vi "Read tau Obs.vi"(8 "error in (no error)":errorcluster, 11 "tCRD in":refnum<class "Aircraft OPCCRD.lvclass">) -> (0 "error out":errorcluster, 2 "tauObs":refnum<class "File Observer.lvclass">, 3 "tCRD out":refnum<class "Aircraft OPCCRD.lvclass">)   [LabVIEW 2015, in "Aircraft OPCCRD.lvclass"]
uses:
  Aircraft OPCCRD.lvclass
  Reusable/File IO/Class/File Observer.lvclass
  Aircraft OPCCRD.lvclass/Aircraft OPCCRD.ctl
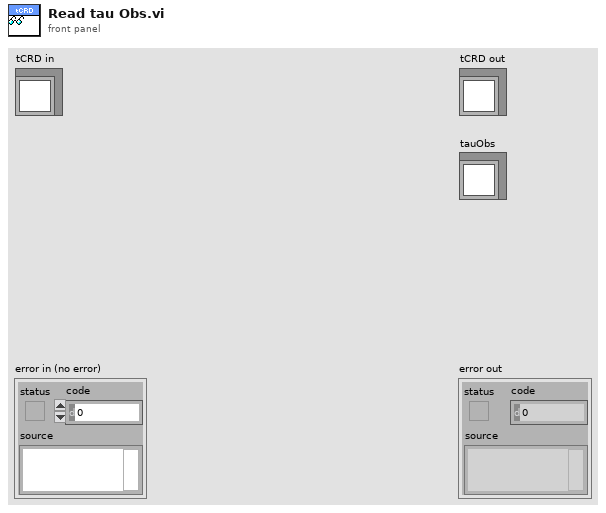
[diagram p1: front panel]
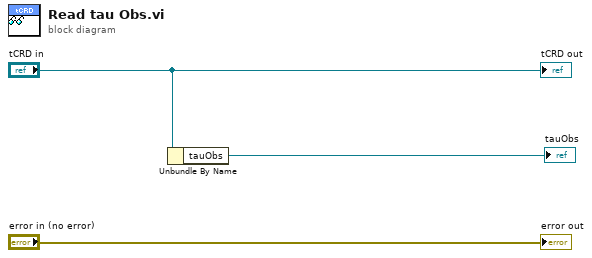
[diagram p0: block diagram]
diagram:
  n1 = Unbundle By Name("tCRD in") -> ("tauObs"=→"tauObs":refnum<class "File Observer.lvclass">)
  "error out" <- "error in (no error)"
  "tCRD out" <- "tCRD in"
